vi "GetTextFromRingCtrl.vi"(11 "enum ref":refnum<vi>) -> (3 "string out":string)   [LabVIEW 2018, in "Library-Ctrl.lvlib"]
uses:
  Library-Ctrl.lvlib
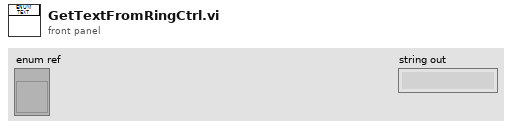
[diagram p1: front panel]
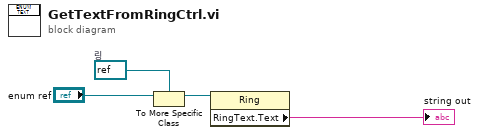
[diagram p0: block diagram]
diagram:
  w3 = refnum<vi> refnum  # 링
  n1 = To More Specific Class(target class=w3, reference="enum ref") -> (specific class reference=w2:refnum<vi>)  [unwired: 1 in, 1 out]
  n2 = property class="Ring"(reference=w2) -> ("RingText.Text"=→"string out":string)  [unwired: 1 in, 2 out]
